vi "Demo.vi"() -> ()   [LabVIEW 2013, in "LV Process library.lvlib"]
uses:
  LV Process library.lvlib
panel:
  out "debug data":T1(array[cluster])
  in  "byte count":i32=1024
  in  "timeout [ms]":i32=10
  in  "write buffer":string="date /T\nexit\n"
  out "read buffer":string
  out "bytes written":i32
  out "exit code":i32
  out "error out":errorcluster
  in  "command":string="cmd"
  in  "working folder":string="c:\\"
  # "What demo does:\n\n1,starts windows command line by \ncommand 'cmd' in working directory 'c:\\',\n\n2. writes commands 'date /T' and 'exit' to stdin,\n\n4, waits 200 ms\n\n3, reads output of stdout,\n\n4, waits 10 ms for process exit\n\n5, if not exited, kills the process\n\n6, clean up handles"
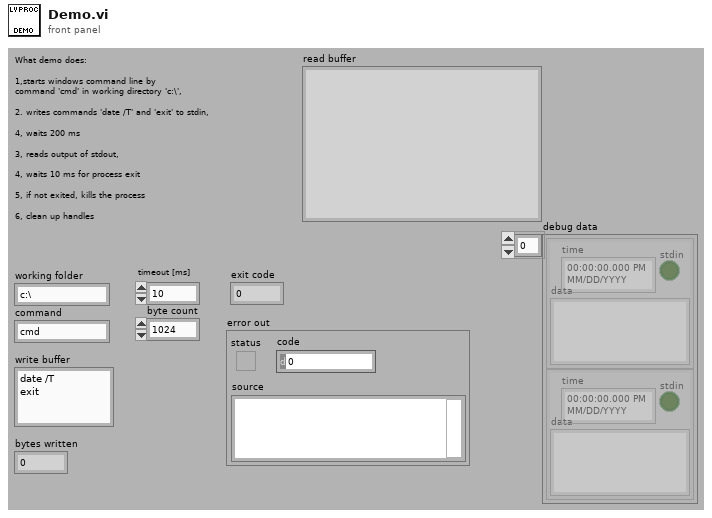
[diagram p1: front panel]
types:
  T1 = cluster{"time":timestamp, "stdin":bool, "data":string}[]
  T2 = typedef "LV Process library.lvlib/Pipe Handle.ctl" = cluster{"lv_proc.dll file path":path, "process instance handle":u32[], "debug mode":bool, "debug data":cluster{"time":timestamp, "stdin":bool, "data":string}[]}
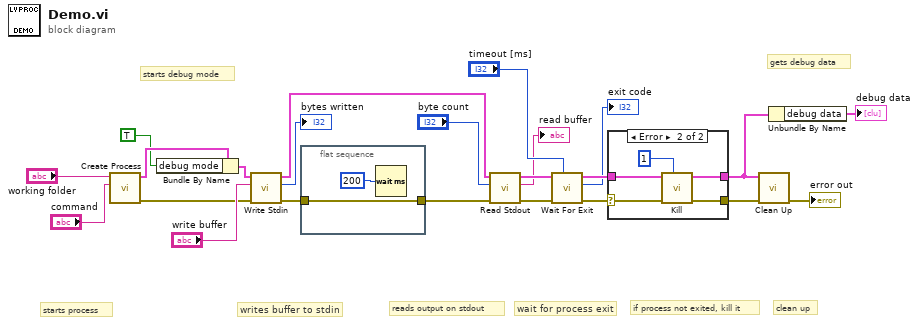
[diagram p0: block diagram]
diagram:
  # "gets debug data"
  # "starts debug mode"
  # "clean up"
  # "if process not exited, kill it"
  # "wait for process exit"
  # "reads output on stdout"
  # "writes buffer to stdin"
  # "starts process"
  n1 = call "Create Process.vi"("command"="command", "working folder"="working folder") -> ("error out"=w8:errorcluster, "pipe handle"=w5:T2)  [unwired: 8 in]
  n2 = Bundle By Name(cluster=w5, "debug mode"=TRUE) -> (w3:T2)
  n3 = call "Write Stdin.vi"("error in"=w8, "write buffer"="write buffer", "pipe in"=w3) -> ("error out"=w6:errorcluster, "return count"=→"bytes written":i32, "pipe out"=w17:T2)  [unwired: 6 in]
  n4 = flat-sequence {
    tunnel: [w24] -> w7
    tunnel: w6 -> [w24]
    frame #0 {
      n5 = Wait (ms)(milliseconds to wait=u32 200) -> ()  [unwired: 1 out]
    }
  }
  n6 = call "Read Stdout.vi"("error in"=w7, "byte count"="byte count", "pipe in"=w17) -> ("error out"=w18:errorcluster, "read buffer"=→"read buffer":string, "pipe out"=w16:T2)  [unwired: 3 in, 3 out]
  n7 = call "Wait For Exit.vi"("timeout [ms]"="timeout [ms]", "error in"=w18, "pipe in"=w16) -> ("error out"=w14:errorcluster, "exit code"=→"exit code":i32, "pipe out"=w20:T2)  [unwired: 6 in]
  n8 = case shown="Error" w14 {
    selector: w14 -> [w26 w28]
    tunnel: w20 -> [w27 w32]
    tunnel: [w26 w29] -> w13
    tunnel: [w27 w30] -> w2
    frame No Error {
    }
    frame Error {
      n9 = call "Kill.vi"("timeout [ms]"=1, "error in"=w28, "pipe in"=w32) -> ("error out"=w29:errorcluster, "pipe out"=w30:T2)  [unwired: 7 in]
    }
  }
  n10 = call "Clean Up.vi"("error in"=w13, "pipe in"=w2) -> ("error out"=→"error out":errorcluster)  [unwired: 9 in]
  n11 = Unbundle By Name(w2) -> ("debug data"=→"debug data":T1)
